vi "Get Events.vi"(0 "Display State In":T2={"Prompt"="Click to add", "Listbox"=refnum, "events"={"Items Changed"=refnum, "List Changed"=refnum}, "allow move"=FALSE}, 9 "Container State":T3, 11 "error in (no error)":errorcluster) -> (4 "Display State Out":T2={"Prompt"="Click to add", "Listbox"=refnum, "events"={"Items Changed"=refnum, "List Changed"=refnum}, "allow move"=FALSE}, 8 "events":T1, 15 "error out":errorcluster)   [LabVIEW 2020, in "KListbox.xctl"]
uses:
  KListbox.xctl
  <vilib>/_xctls/Container State.ctl
  State.ctl
  Events.ctl
  Event Action.ctl
  <vilib>/_xctls/XControlSupport.lvlib
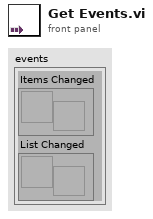
[diagram p1: front panel]
types:
  T1 = typedef "KListbox.xctl/Events.ctl" = cluster{"Items Changed":refnum<user-event>, "List Changed":refnum<user-event>}
  T2 = typedef "KListbox.xctl/State.ctl" = cluster{"Prompt":string, "Listbox":refnum<vi>, "events":T1, "allow move":bool}
  T3 = typedef "XControlSupport.lvlib/Container State.ctl" = cluster{"Indicator?":bool, "Run Mode?":bool, " Refnum":refnum<vi>}
  T4 = typedef "KListbox.xctl/Event Action.ctl" = enum16{"Select", "Add", "Delete", "Edit"}
  T5 = cluster{"Data":refnum<user-event>, "Data":refnum<user-event>}
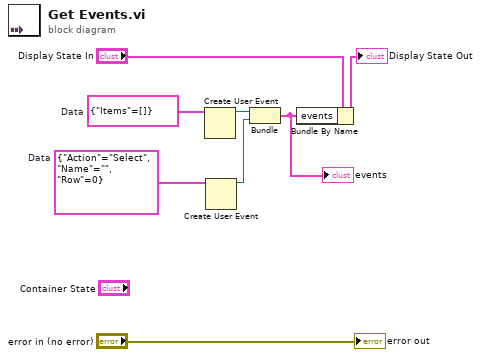
[diagram p0: block diagram]
diagram:
  w3 = cluster{"Action":T4, "Name":string, "Row":i32} {"Action"=enum."Select", "Name"="", "Row"=0}  # Data
  w4 = cluster{"Items":string[]} {"Items"=[]}  # Data
  n1 = Create User Event(user event datatype=w4) -> (user event=w6:refnum<user-event>)  [unwired: 1 in, 1 out]
  n2 = Create User Event(user event datatype=w3) -> (user event=w5:refnum<user-event>)  [unwired: 1 in, 1 out]
  n3 = Bundle("Data"=w6, "Data"=w5) -> (w1:T5)  [unwired: 1 in]
  "events" <- w1
  n4 = Bundle By Name(cluster="Display State In", "events"=w1) -> (→"Display State Out":T2)
  "error out" <- "error in (no error)"
